vi "Testpath.vi"() -> ()   [LabVIEW 2016]
panel:
  out "Path":path
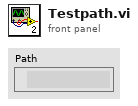
[diagram p1: front panel]
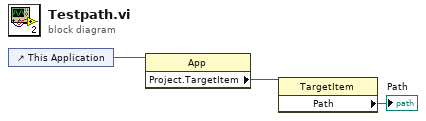
[diagram p0: block diagram]
diagram:
  n1 = control-ref of="This Application"() -> (w3:refnum<vi>)
  n2 = property class="App"(reference=w3) -> ("Project.TargetItem"=w2:refnum<vi>)  [unwired: 1 in, 2 out]
  n3 = property class="TargetItem"(reference=w2) -> ("Path"=→"Path":path)  [unwired: 1 in, 2 out]
